vi "SetDoubleTaskVariables.vi"(6 "values":dbl[](array[numeric]), 8 "error in (no error)":errorcluster, 9 "varNumber":i32, 10 "taskId":i32(ring) items=["TLibrary", "T01", "T02", "T03", "T04", "T05", "T06", "T07", "T08", "T09", "T10", "T11", "T12", "T13", "T14", "T15", "T16", "T17", "T18", "T19", "T20", "T21", "T22", "T23", "T24", "T25", "T26", "T27", "T28", "T29", "T30", "T31"], 11 "controller in":refnum<k24>) -> (0 "error out":errorcluster, 3 "controller out":refnum<k24>)   [LabVIEW 2020, in "Aerotech.lvlib"]
uses:
  Aerotech.lvlib
  C:/Users/HEP/Documents/GitHub/UCSB-Gantry-HEP/Drivers/Aerotech A3200/Bin/Aerotech.A3200.LabVIEW.dll
  UCSB-Gantry-HEP/Drivers/Aerotech A3200/Bin/Aerotech.A3200.LabVIEW.dll
  C:/Program Files (x86)/Aerotech/A3200/LabVIEW/2010/Bin/Aerotech.A3200.dll
  Program Files (x86)/Aerotech/A3200/LabVIEW/2010/Bin/Aerotech.A3200.dll
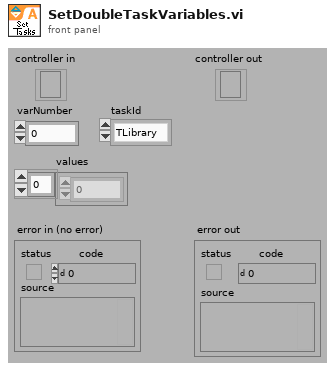
[diagram p1: front panel]
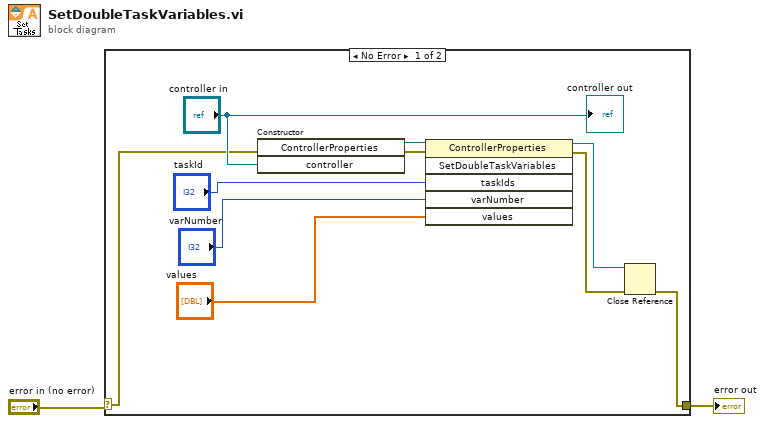
[diagram p0: block diagram]
diagram:
  n1 = case shown="No Error" "error in (no error)" {
    selector: "error in (no error)" -> [w11 w13]
    tunnel: [w3 w13] -> w1
    frame No Error {
      n2 = constructor class="ControllerProperties"(error in=w11, "controller"="controller in") -> (reference out=w10:refnum<k24>, error out=w9:errorcluster)  [unwired: 2 in, 2 out]
      n3 = invoke class="ControllerProperties" method="SetDoubleTaskVariables"(reference=w10, error in=w9, "taskIds"="taskId", "varNumber"="varNumber", "values"="values") -> (reference out=w5:refnum<k24>, error out=w4:errorcluster)  [unwired: 1 in, 4 out]
      n4 = Close Reference(reference=w5, error in (no error)=w4) -> (error out=w3:errorcluster)
      "controller out" <- "controller in"
    }
    frame Error {
    }
  }
  "error out" <- w1
